vi "GET_security_access_status.vi"(8 "API Key":string="cheia04042025tema2restfulapi") -> (1 "headers":string, 2 "body":string, 3 "error out get":errorcluster)   [LabVIEW 2024]
uses:
  <vilib>/httpClient/LabVIEWHTTPClient.lvlib
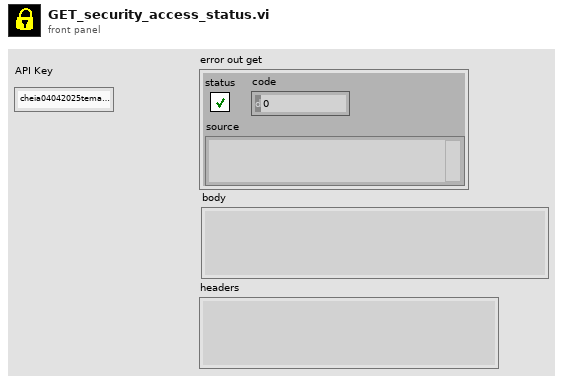
[diagram p1: front panel]
types:
  T1 = typedef "LabVIEWHTTPClient.lvlib/ClientHandle.ctl" = refnum<k1>
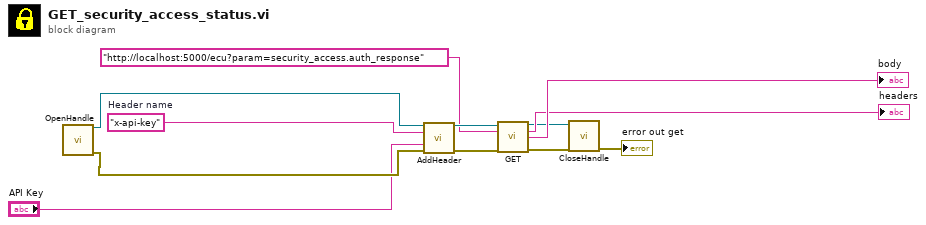
[diagram p0: block diagram]
diagram:
  w3 = "x-api-key"  # Header name
  n1 = call <vilib>:"OpenHandle.vi"() -> ("client handle out"=w4:T1, "error out"=w5:errorcluster)  [unwired: 14 in]
  n2 = call <vilib>:"AddHeader.vi"("client handle"=w4, "header"=w3, "value"="API Key", "error in (no error)"=w5) -> ("client handle out"=w7:T1, "error out"=w6:errorcluster)  [unwired: 10 in]
  n3 = call <vilib>:"GET.vi"("client handle"=w7, "url"="http://localhost:5000/ecu?param=security_access.auth_response", "error in (no error)"=w6) -> ("client handle out"=w9:T1, "headers"=→"headers":string, "body"=→"body":string, "error out"=w8:errorcluster)  [unwired: 9 in]
  n4 = call <vilib>:"CloseHandle.vi"("client handle"=w9, "error in (no error)"=w8) -> ("error out"=→"error out get":errorcluster)  [unwired: 13 in]
